vi "Tote Winch Interface.vi"(11 "Winch Command":T1(ring)=enum."Hold") -> ()   [LabVIEW 2014]
panel:
  out "Actual Height":dbl=8.15222954425 format="%#_5f"
  in  "Winch Assembly mechanical Offset":dbl=8.0605
  out "Raw Encoder Distance":dbl=0.09172954425 format="%#_4f"
  in  "Hovering 2nd Tote":dbl=22.462
  in  "Stacked 2nd Tote":dbl=16.996
  in  "Ground":dbl=8.2
  in  "Scoring Platform":dbl=11.971
  out "Lower Limit Reached":bool
  out "Upper Limit Reached":bool
  in  "Desired Height":dbl
  out "Drive Output":dbl=0.047770455749999385 format="%#_4f"
  in  "Kp":dbl=1.0
  in  "Reset Encoder?":bool
  out "Stopped":bool=TRUE
  out "Rate":dbl format="%#_4f"
  out "Direction":bool=TRUE
  in  "Max Winch Drive Torque":dbl=1.0 format="%#_13g"
  # "+"
  # "="
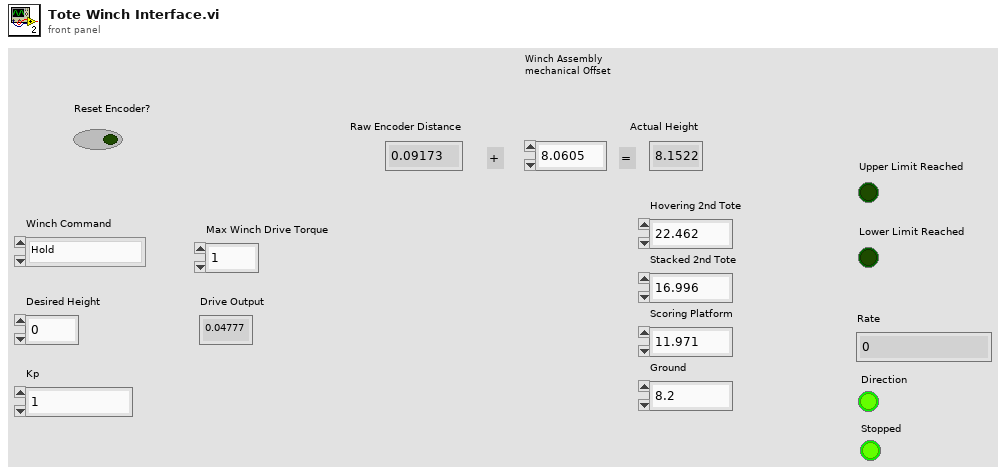
[diagram p1: front panel]
types:
  T1 = enum16{"Off", "Hold", "Jog Down", "Jog Up", "Ground", "Scoring Platform", "Stacked 2nd Tote", "Hovering 2nd Tote"}
  T2 = typedef "WPI_DigitalInputDevRef.ctl" = cluster{"DevStatus":errorcluster, "DIO Channel":T3, "Controller":T4}
  T3 = typedef "FPGA_DIOChannel.ctl" = enum8{"DIO 0", "DIO 1", "DIO 2", "DIO 3", "DIO 4", "DIO 5", "DIO 6", "DIO 7", "DIO 8", "DIO 9", "DIO MXP 0", "DIO MXP 1", "DIO MXP 2", "DIO MXP 3", "DIO MXP 4", "DIO MXP 5", "DIO MXP 6", "DIO MXP 7", "DIO MXP 8", "DIO MXP 9", "DIO MXP 10", "DIO MXP 11", "DIO MXP 12", "DIO MXP 13", "DIO MXP 14", "DIO MXP 15", "Invalid"}
  T4 = typedef "FPGA_TypedefDigitalModule.ctl" = enum16{"Controller 1"}
  T5 = typedef "WPI_EncoderDevRef.ctl" = cluster{"DevStatus":errorcluster, "EncoderIndex":T6, "CounterIndex":T7, "DistancePerCount":dbl, "Decoding Type":T8}
  T6 = typedef "FPGA_EncoderIdx.ctl" = enum8{"Enc 0", "Enc 1", "Enc 2", "Enc 3", "Enc 4", "Enc 5", "Enc 6", "Enc 7", "Invalid"}
  T7 = typedef "FPGA_CounterCtrSystemIndex.ctl" = enum8{"Ctr 0", "Ctr 1", "Ctr 2", "Ctr 3", "Ctr 4", "Ctr 5", "Ctr 6", "Ctr 7", "Invalid"}
  T8 = typedef "WPI_EncoderType.ctl" = enum16{"1x", "2x", "4x"}
  T9 = enum16{"Control Off", "Control Hold", "Control Jog Up", "Control Jog Down"}
  T10 = typedef "WPI_MotorControlDeviceRef.ctl" = cluster{"DeviceStatus":errorcluster, "Type":T11, "PWM":cluster{"Controller":T4, "PWM Channel":T12, "DeadBand":T13}, "CAN":cluster{"Device Number":u8, "Control Mode":T14, "Semaphore":T15, "Max Vout":dbl, "TalonSRX Control Mode":T16}, "Invert":bool, "TransformRef":T17, "InvTransformRef":T17}
  T11 = typedef "WPI_MotorControlType.ctl" = enum16{"PWM", "CAN", "CANTalonSRX"}
  T12 = typedef "FPGA_DIOPWMChannel.ctl" = enum8{"PWM 0", "PWM 1", "PWM 2", "PWM 3", "PWM 4", "PWM 5", "PWM 6", "PWM 7", "PWM 8", "PWM 9", "PWM MXP 0", "PWM MXP 1", "PWM MXP 2", "PWM MXP 3", "PWM MXP 4", "PWM MXP 5", "PWM MXP 6", "PWM MXP 7", "PWM MXP 8", "PWM MXP 9", "Invalid"}
  T13 = typedef "WPI_PWMDeadband.ctl" = cluster{"Name":string, "maxPositivePwm":i32, "minPositivePwm":i32, "centerPwm":i32, "maxNegativePwm":i32, "minNegativePwm":i32, "angularRange":u16}
  T14 = typedef "WPI_CANJaguar_ControlMode.ctl" = enum8{"Percent VBus", "Current", "Speed", "Position", "Voltage"}
  T15 = typedef "Semaphore RefNum" = refnum<k1>
  T16 = typedef "WPI_CANTalonSRX_APIControlMode.ctl" = enum8{"Percent VBus", "Speed", "Position", "Slave", "Unchanged / Invalid"}
  T17 = typedef "WPI_PWMTransform_ConPane.ctl" = refnum<vi>
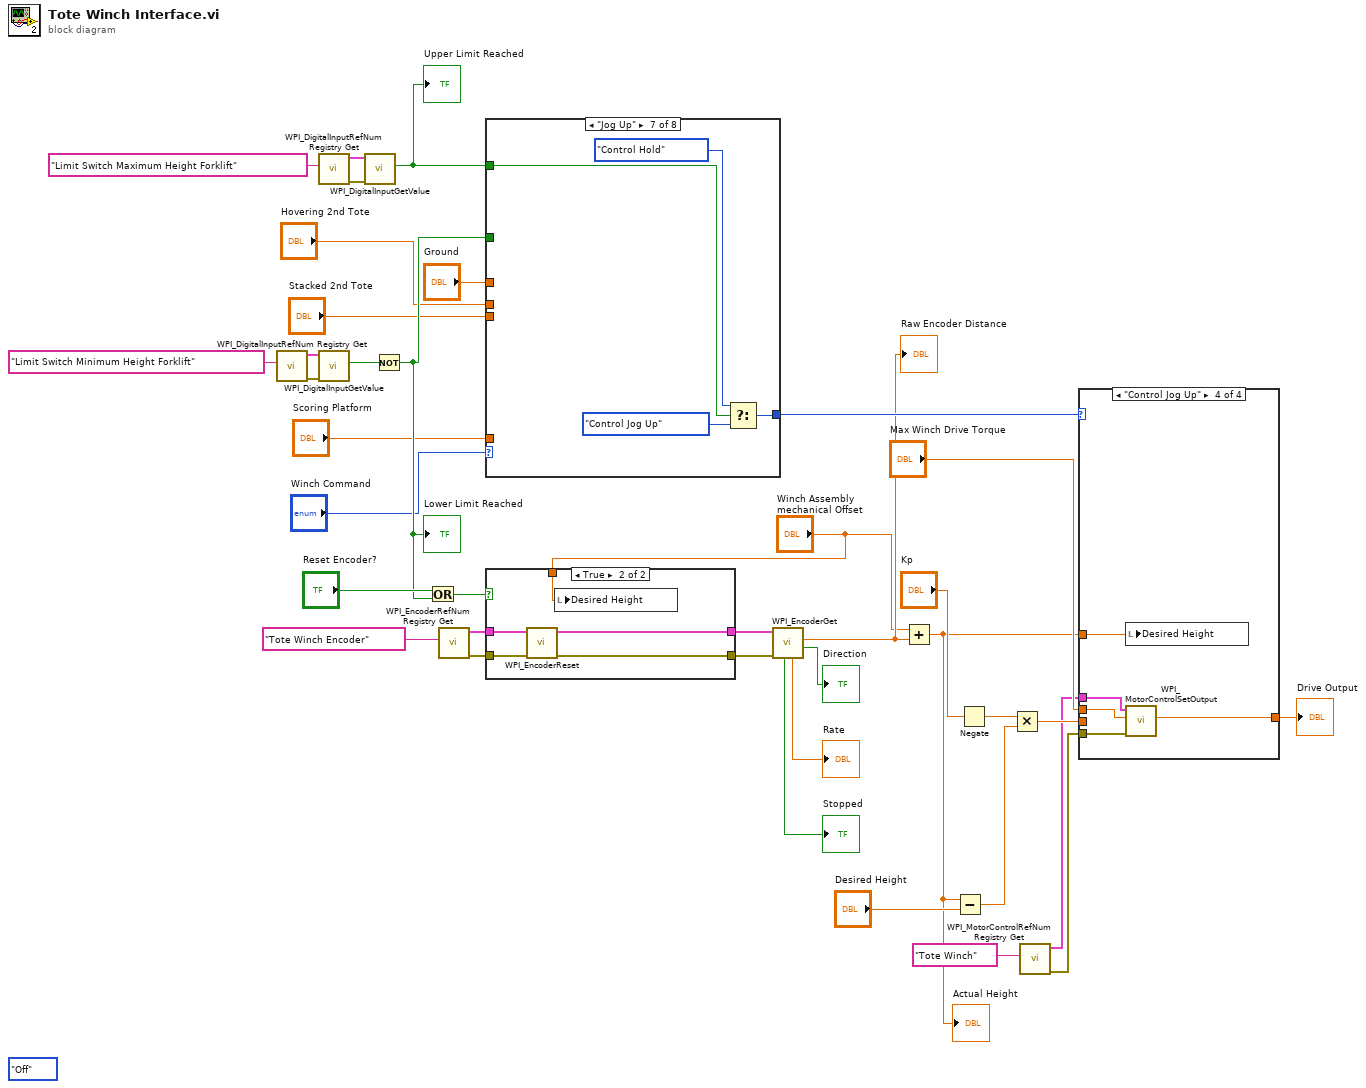
[diagram p0: block diagram]
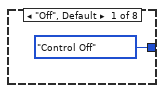
[diagram p2: hidden frame]
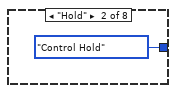
[diagram p3: hidden frame]
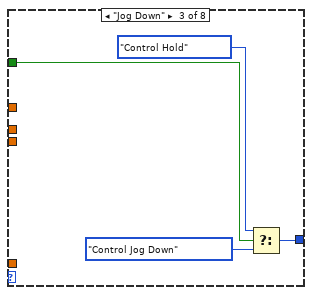
[diagram p4: hidden frame]
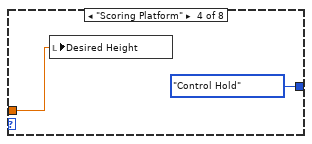
[diagram p5: hidden frame]
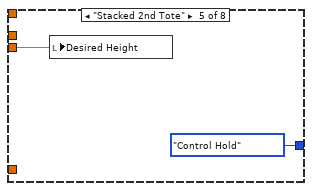
[diagram p6: hidden frame]
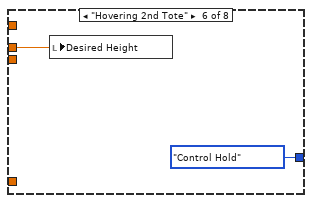
[diagram p7: hidden frame]
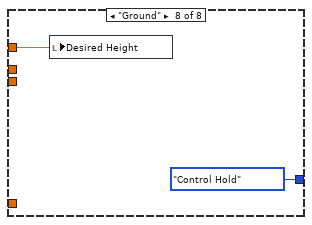
[diagram p8: hidden frame]
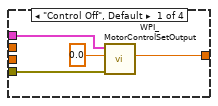
[diagram p10: hidden frame]
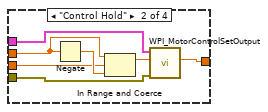
[diagram p11: hidden frame]
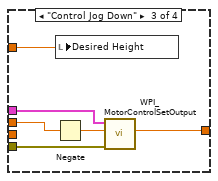
[diagram p12: hidden frame]
diagram:
  (unwired) enum16{"Off", "Hold", "Jog Up", "Jog Down"}."Off"
  n1 = call <vilib>:"WPI_DigitalInputRefNum Registry Get.vi"("refnum name"="Limit Switch Minimum Height Forklift") -> ("error out"=w21:errorcluster, "DigitalInputDevRef"=w22:T2)  [unwired: 9 in]
  n2 = call <vilib>:"WPI_DigitalInputRefNum Registry Get.vi"("refnum name"="Limit Switch Maximum Height Forklift") -> ("error out"=w15:errorcluster, "DigitalInputDevRef"=w16:T2)  [unwired: 9 in]
  n3 = call <vilib>:"WPI_DigitalInputGetValue.vi"("error in (no error)"=w21, "DigitalInputDevRef"=w22) -> ("Value"=w12:bool)  [unwired: 7 in, 2 out]
  n4 = call <vilib>:"WPI_DigitalInputGetValue.vi"("error in (no error)"=w15, "DigitalInputDevRef"=w16) -> ("Value"=w13:bool)  [unwired: 7 in, 2 out]
  "Upper Limit Reached" <- w13
  n5 = Not(x=w12) -> (.not. x?=w11:bool)
  "Lower Limit Reached" <- w11
  n6 = Or(x="Reset Encoder?", y=w11) -> (x .or. y?=w18:bool)
  n7 = call <vilib>:"WPI_EncoderRefNum Registry Get.vi"("refnum name"="Tote Winch Encoder") -> ("error out"=w32:errorcluster, "EncoderDevRef"=w33:T5)  [unwired: 9 in]
  n8 = case shown="\"Jog Up\"" "Winch Command" {
    tunnel: [T9."Control Off" T9."Control Hold" w44 T9."Control Hold" T9."Control Hold" T9."Control Hold" w54 T9."Control Hold"] -> w5
    tunnel: w11 -> [_ _ w43 _ _ _ _ _]
    tunnel: w13 -> [_ _ _ _ _ _ w53 _]
    tunnel: "Scoring Platform" -> [_ _ _ w46 _ _ _ _]
    tunnel: "Stacked 2nd Tote" -> [_ _ _ _ w48 _ _ _]
    tunnel: "Hovering 2nd Tote" -> [_ _ _ _ _ w50 _ _]
    tunnel: "Ground" -> [_ _ _ _ _ _ _ w56]
    frame "Off", Default {
    }
    frame "Hold" {
    }
    frame "Jog Down" {
      n9 = Select(t=T9."Control Hold", s=w43, f=T9."Control Jog Down") -> (s? t:f=w44:T9)
    }
    frame "Scoring Platform" {
      n10 = local write "Desired Height"(w46) -> ()
    }
    frame "Stacked 2nd Tote" {
      n11 = local write "Desired Height"(w48) -> ()
    }
    frame "Hovering 2nd Tote" {
      n12 = local write "Desired Height"(w50) -> ()
    }
    frame "Jog Up" {
      n13 = Select(t=T9."Control Hold", s=w53, f=T9."Control Jog Up") -> (s? t:f=w54:T9)
    }
    frame "Ground" {
      n14 = local write "Desired Height"(w56) -> ()
    }
  }
  n15 = case shown="True" w18 {
    tunnel: w33 -> [w58 w63]
    tunnel: w32 -> [w57 w62]
    tunnel: [w57 w61] -> w31
    tunnel: [w58 w60] -> w30
    tunnel: "Winch Assembly mechanical Offset" -> [_ w59]
    frame False {
    }
    frame True {
      n16 = call <vilib>:"WPI_EncoderReset.vi"("error in (no error)"=w62, "EncoderDevRef"=w63) -> ("error out"=w61:errorcluster, "EncoderDevRef"=w60:T5)  [unwired: 8 in]
      n17 = local write "Desired Height"(w59) -> ()
    }
  }
  n18 = call <vilib>:"WPI_EncoderGet.vi"("error in (no error)"=w31, "EncoderDevRef"=w30) -> ("Direction"=→"Direction":bool, "Distance"=w3:dbl, "Rate"=→"Rate":dbl, "Stopped"=→"Stopped":bool)  [unwired: 4 in, 2 out]
  "Raw Encoder Distance" <- w3
  n19 = Add(x="Winch Assembly mechanical Offset", y=w3) -> (x+y=w2:dbl)
  "Actual Height" <- w2
  n20 = Subtract(x=w2, y="Desired Height") -> (x-y=w27:dbl)
  n21 = Negate(x="Kp") -> (-x=w4:dbl)
  n22 = Multiply(x=w4, y=w27) -> (x*y=w25:dbl)
  n23 = call <vilib>:"WPI_MotorControlRefNum Registry Get.vi"("refnum name"="Tote Winch") -> ("error out"=w23:errorcluster, "MotorControlDevRef"=w24:T10)  [unwired: 9 in]
  n24 = case shown="\"Control Jog Up\"" w5 {
    tunnel: "Max Winch Drive Torque" -> [_ w72 w79 w85]
    tunnel: w24 -> [w66 w74 w78 w84]
    tunnel: w23 -> [w65 w73 w77 w83]
    tunnel: w25 -> [_ w70 _ _]
    tunnel: w2 -> [_ _ w76 w82]
    tunnel: [w64 w68 w75 w81] -> w17
    frame "Control Off", Default {
      n25 = call <vilib>:"WPI_MotorControlSetOutput.vi"("error in (no error)"=w65, "Output"=0.0 ("Motor Output"), "MotorControlDevRef"=w66) -> ("Motor Output"=w64:dbl)  [unwired: 6 in, 2 out]
    }
    frame "Control Hold" {
      n26 = Negate(x=w72) -> (-x=w71:dbl)
      n27 = In Range and Coerce(upper limit=w72, x=w70, lower limit=w71) -> (coerced(x)=w69:dbl)  [unwired: 1 out]
      n28 = call <vilib>:"WPI_MotorControlSetOutput.vi"("error in (no error)"=w73, "Output"=w69, "MotorControlDevRef"=w74) -> ("Motor Output"=w68:dbl)  [unwired: 6 in, 2 out]
    }
    frame "Control Jog Down" {
      n29 = Negate(x=w79) -> (-x=w80:dbl)
      n30 = local write "Desired Height"(w76) -> ()
      n31 = call <vilib>:"WPI_MotorControlSetOutput.vi"("error in (no error)"=w77, "Output"=w80, "MotorControlDevRef"=w78) -> ("Motor Output"=w75:dbl)  [unwired: 6 in, 2 out]
    }
    frame "Control Jog Up" {
      n32 = local write "Desired Height"(w82) -> ()
      n33 = call <vilib>:"WPI_MotorControlSetOutput.vi"("error in (no error)"=w83, "Output"=w85, "MotorControlDevRef"=w84) -> ("Motor Output"=w81:dbl)  [unwired: 6 in, 2 out]
    }
  }
  "Drive Output" <- w17
